vi "to json string.vi"(8 "error in (no error)":errorcluster, 11 "DSFConfiguration":refnum<class "DSFConfiguration.lvclass">) -> (0 "error out":errorcluster, 2 "JSON string":string)   [LabVIEW 2017, in "DSFConfiguration.lvclass"]
uses:
  DSFConfiguration.lvclass
  Controls/dsf transfer.ctl
  Controls/dsf channel.ctl
  Controls/dsf settings.ctl
  DSFConfiguration.lvclass/DSFConfiguration.ctl
  IDable/IDable.lvclass/IDable.ctl
  DSFPluginSettings/DSFPluginSettings.lvclass/DSFPluginSettings.ctl
  DSFChannel/DSFChannel.lvclass/DSFChannel.ctl
  DSFTransfer/DSFTransfer.lvclass/DSFTransfer.ctl
  IDable/Read id.vi
  DSFPluginSettings/Read plugin settings info.vi
  DSFChannel/Read channel info.vi
  DSFTransfer/Read transfer info.vi
  Read plugins.vi
  Read groups.vi
  Read transfers.vi
  Read channels.vi
  Read settings.vi
  DSFPluginSettings/DSFPluginSettings.lvclass
  C:/github/data-sharing-framework/Source/Configuration API/Classes/IDable/IDable.lvclass
  DSFChannel/DSFChannel.lvclass
  DSFTransfer/DSFTransfer.lvclass
  DSFPlugin/DSFPlugin.lvclass
  DSFGroup/DSFGroup.lvclass
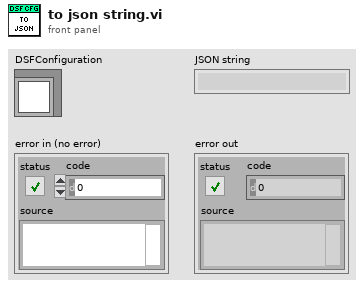
[diagram p1: front panel]
types:
  T1 = typedef "dsf transfer.ctl" = cluster{"byte order":i32, "channel ids":string[], "settings id":string}
  T2 = typedef "dsf channel.ctl" = cluster{"count":i32, "offset":i32, "data type":i32, "vs channel path":string, "settings id":string}
  T3 = typedef "dsf settings.ctl" = cluster{"key":string, "value":string}[]
  T4 = cluster{"transfers":cluster{"id":string, "values":T1}[], "channels":cluster{"id":string, "values":T2}[], "settings":cluster{"id":string, "values":T3}[]}
  T5 = cluster{"accessors:id":string, "accessors:transfer info":T1}
  T6 = cluster{"accessors:id":string, "accessors:channel info":T2}
  T7 = cluster{"accessors:id":string, "accessors:plugin settings info":T3}
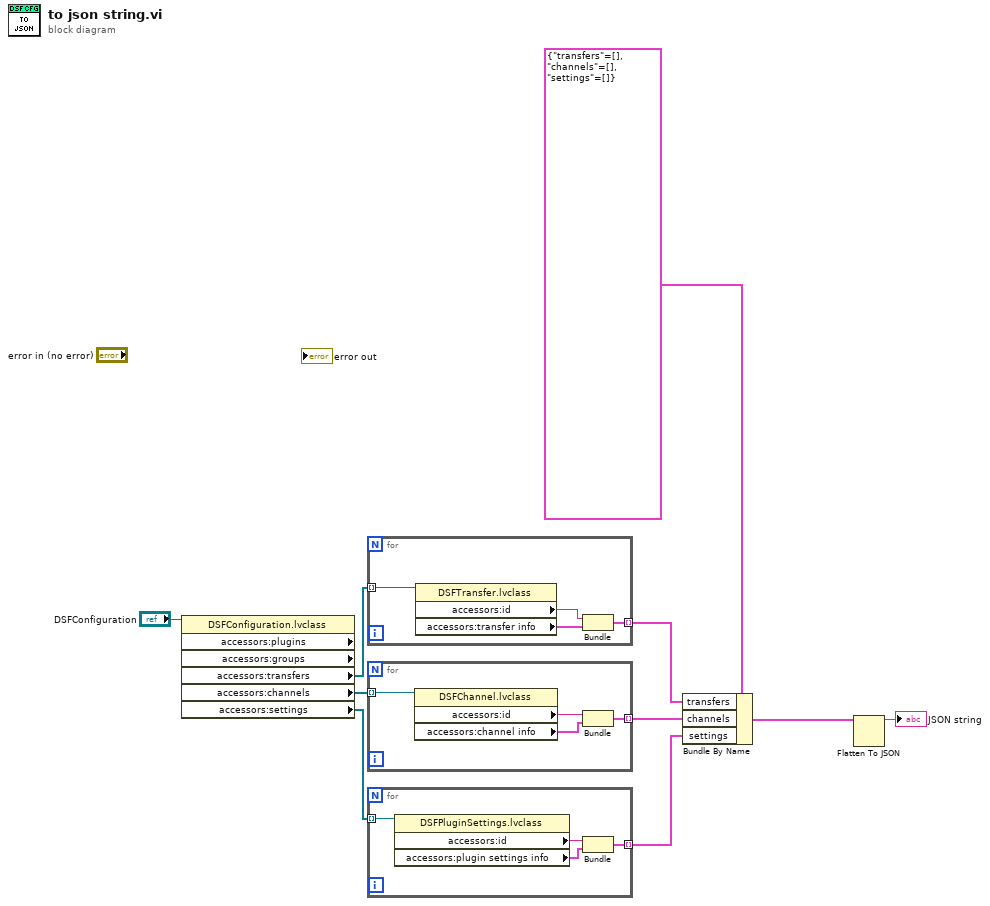
[diagram p0: block diagram]
diagram:
  n1 = property class="DSFConfiguration.lvclass" props=["accessors:plugins", "accessors:groups", "accessors:transfers", "accessors:channels", "accessors:settings"](reference="DSFConfiguration") -> ("accessors:transfers"=w2:refnum<class "DSFTransfer.lvclass">[], "accessors:channels"=w4:refnum<class "DSFChannel.lvclass">[], "accessors:settings"=w3:refnum<class "DSFPluginSettings.lvclass">[])  [unwired: 1 in, 4 out]
  n2 = for {
    tunnel: w2 -> [w14] mode=indexing
    tunnel: [w11] -> w1 mode=indexing
    n3 = property class="DSFTransfer.lvclass"(reference=w14) -> ("accessors:id"=w13:string, "accessors:transfer info"=w12:T1)  [unwired: 1 in, 2 out]
    n4 = Bundle("accessors:id"=w13, "accessors:transfer info"=w12) -> (w11:T5)  [unwired: 1 in]
  }
  n5 = for {
    tunnel: w4 -> [w18] mode=indexing
    tunnel: [w15] -> w6 mode=indexing
    n6 = property class="DSFChannel.lvclass"(reference=w18) -> ("accessors:id"=w17:string, "accessors:channel info"=w16:T2)  [unwired: 1 in, 2 out]
    n7 = Bundle("accessors:id"=w17, "accessors:channel info"=w16) -> (w15:T6)  [unwired: 1 in]
  }
  n8 = for {
    tunnel: [w21] -> w5 mode=indexing
    tunnel: w3 -> [w20] mode=indexing
    n9 = property class="DSFPluginSettings.lvclass"(reference=w20) -> ("accessors:id"=w22:string, "accessors:plugin settings info"=w19:T3)  [unwired: 1 in, 2 out]
    n10 = Bundle("accessors:id"=w22, "accessors:plugin settings info"=w19) -> (w21:T7)  [unwired: 1 in]
  }
  n11 = Bundle By Name(cluster=T4 {"transfers"=[], "channels"=[], "settings"=[]}, "transfers"=w1, "channels"=w6, "settings"=w5) -> (w7:T4)
  n12 = Flatten To JSON(anything=w7) -> (JSON string=→"JSON string":string)  [unwired: 2 in, 1 out]
